vi "Init DAQ (In) Single Channel.vi"(8 "error in (no error)":errorcluster, 10 "Trigger Channel (Find Using NI Max)":tag="Dev1/ai16", 11 "Timing":T1={"Sampling Rate (Hz)"=1000.0, "Display Rate (Hz)"=100.0, "Sampling Mode"=2} {"Sampling Mode" items=["Finite Samples", "Continuous Samples", "Hardware Timed Single Point"]; "Sampling Rate (Hz)" format="%0.2f"}) -> (0 "error out":errorcluster, 2 "Channel Array":refnum<k21>[](array[refnum]))   [LabVIEW 2017]
uses:
  Controls/Timing Controls.ctl
  <vilib>/DAQmx/create/channels.llb/DAQmx Create Channel (AI-Voltage-Basic).vi
  <vilib>/DAQmx/configure/timing.llb/DAQmx Timing (Sample Clock).vi
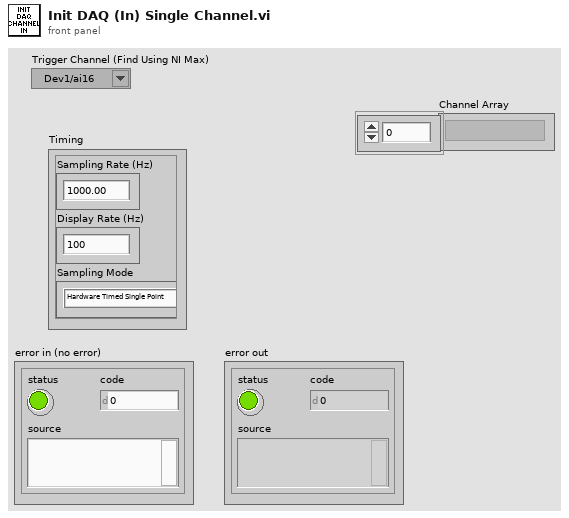
[diagram p1: front panel]
types:
  T1 = typedef "Timing Controls.ctl" = cluster{"Sampling Rate (Hz)":dbl, "Display Rate (Hz)":dbl, "Sampling Mode":i32}
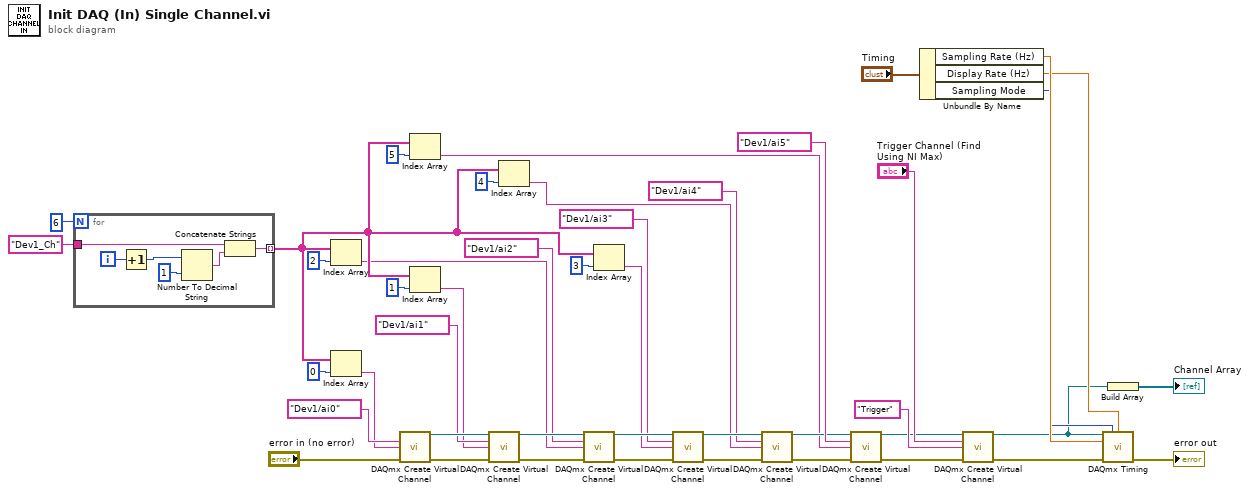
[diagram p0: block diagram]
diagram:
  n1 = for {
    N: 6 -> [_]
    tunnel: "Dev1_Ch" ("name to assign") -> [w46]
    tunnel: [w45] -> w11 mode=indexing
    i -> [w50]
    n2 = Increment(x=w50) -> (x+1=w48:i32)
    n3 = Number To Decimal String(number=w48, width (-)=i16 1) -> (decimal integer string=w47:string)
    n4 = Concatenate Strings(w46, w47) -> (w45:string)
  }
  n5 = Index Array(array=w11, index=2) -> (element=w9:string)
  n6 = Index Array(array=w11, index=0) -> (element=w17:string)
  n7 = call-poly <vilib>:"DAQmx Create Virtual Channel.vi"("physical channels"=tag "Dev1/ai0", "name to assign"=w17, "error in"="error in (no error)") -> ("task out"=w36:refnum<k21>, "error out"=w32:errorcluster)  [unwired: 11 in]
  n8 = Index Array(array=w11, index=5) -> (element=w6:string)
  n9 = Index Array(array=w11, index=1) -> (element=w10:string)
  n10 = call-poly <vilib>:"DAQmx Create Virtual Channel.vi"("task in"=w36, "physical channels"=tag "Dev1/ai1", "name to assign"=w10, "error in"=w32) -> ("task out"=w34:refnum<k21>, "error out"=w30:errorcluster)  [unwired: 10 in]
  n11 = Index Array(array=w11, index=4) -> (element=w7:string)
  n12 = call-poly <vilib>:"DAQmx Create Virtual Channel.vi"("task in"=w34, "physical channels"=tag "Dev1/ai2", "name to assign"=w9, "error in"=w30) -> ("task out"=w33:refnum<k21>, "error out"=w28:errorcluster)  [unwired: 10 in]
  n13 = Index Array(array=w11, index=3) -> (element=w8:string)
  n14 = call-poly <vilib>:"DAQmx Create Virtual Channel.vi"("task in"=w33, "physical channels"=tag "Dev1/ai3", "name to assign"=w8, "error in"=w28) -> ("task out"=w25:refnum<k21>, "error out"=w26:errorcluster)  [unwired: 10 in]
  n15 = call-poly <vilib>:"DAQmx Create Virtual Channel.vi"("task in"=w25, "physical channels"=tag "Dev1/ai4", "name to assign"=w7, "error in"=w26) -> ("task out"=w22:refnum<k21>, "error out"=w21:errorcluster)  [unwired: 10 in]
  n16 = call-poly <vilib>:"DAQmx Create Virtual Channel.vi"("task in"=w22, "physical channels"=tag "Dev1/ai5", "name to assign"=w6, "error in"=w21) -> ("task out"=w4:refnum<k21>, "error out"=w5:errorcluster)  [unwired: 10 in]
  n17 = Unbundle By Name("Timing") -> ("Sampling Rate (Hz)"=w39:dbl, "Display Rate (Hz)"=w38:dbl, "Sampling Mode"=w37:i32)
  n18 = call-poly <vilib>:"DAQmx Create Virtual Channel.vi"("task in"=w4, "physical channels"="Trigger Channel (Find Using NI Max)", "name to assign"="Trigger", "error in"=w5) -> ("task out"=w1:refnum<k21>, "error out"=w2:errorcluster)  [unwired: 10 in]
  n19 = call-poly <vilib>:"DAQmx Timing.vi"("task/channels in"=w1, "sample mode"=w37, "samples per channel"=w38, "rate"=w39, "error in"=w2) -> ("error out"=→"error out":errorcluster)  [unwired: 9 in, 1 out]
  n20 = Build Array(w1) -> (→"Channel Array":refnum<k21>[])
